vi "CRC_Calc.vi"(11 "Data_in":u8[](array[numeric])) -> (3 "CRC":u8 format="%x")   [LabVIEW 2023, in "LP_CRC.lvlib"]
uses:
  LP_CRC.lvlib
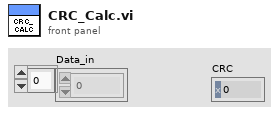
[diagram p1: front panel]
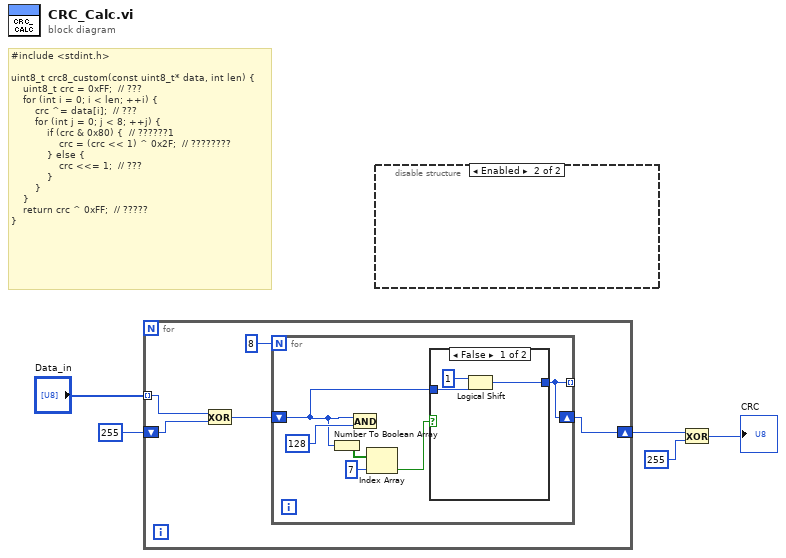
[diagram p0: block diagram]
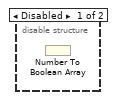
[diagram p2: hidden frame]
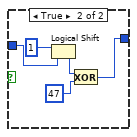
[diagram p3: hidden frame]
diagram:
  # "#include <stdint.h>\n\nuint8_t crc8_custom(const uint8_t* data, int len) {\n    uint8_t crc = 0xFF;  // ???\n    for (int i = 0; i < len; ++i) {\n        crc ^= data[i];  // ???\n        for (int j = 0; j < 8; ++j) {\n            if (crc & 0x80) {  // ??????1\n                crc = (crc << 1) ^ 0x2F;  // ????????\n            } else {\n                crc <<= 1;  // ???\n            }\n        }\n    }\n    return crc ^ 0xFF;  // ?????\n}"
  n1 = for {
    tunnel: "Data_in" -> [w8] mode=indexing
    shift-right: [w9] -> w4
    shift-left: u8 255 ("Numeric") -> [w7]
    n2 = Exclusive Or(1:w7, 2:w8) -> (0:w6:u8)
    n3 = for {
      N: 8 -> [_]
      shift-right: [w11] -> w9
      shift-left: w6 -> [w15]
      tunnel: [w11] -> _ mode=indexing
      n4 = Number To Boolean Array(number=w15) -> (Boolean array=w14:bool[])
      n5 = And(x=w15, y=u8 128) -> ()  [unwired: 1 out]
      n6 = Index Array(array=w14, index=7) -> (element=w12:bool)
      n7 = case shown="False" w12 {
        tunnel: w15 -> [w18 w23]
        tunnel: [w17 w20] -> w11
        frame False {
          n8 = Logical Shift(y=i16 1, x=w18) -> (x << y=w17:u8)
        }
        frame True {
          n9 = Logical Shift(y=i16 1, x=w23) -> (x << y=w22:u8)
          n10 = Exclusive Or(1:u8 47 ("y"), 2:w22) -> (0:w20:u8)
        }
      }
    }
  }
  n11 = disable-structure shown="Enabled" {
    frame Disabled {
      n12 = Number To Boolean Array() -> ()  [unwired: 1 in, 1 out]
    }
    frame Enabled {
    }
  }
  n13 = Exclusive Or(1:u8 255 ("Numeric"), 2:w4) -> (0:→"CRC":u8)
